vi "Framework Configuration 1.1 Finalize.vi"(8 "error in (no error)":errorcluster, 10 "dsf version (1.1)":T1={"major"=1, "minor"=1, "fix"=0, "build"=""}, 11 "framework configuration 1.1":T2) -> (0 "error out":errorcluster, 2 "final dsf version":T1, 3 "dsf configuration json":string)   [LabVIEW 2017, in "DSF Core.lvlib" / "Configuration Session.lvclass"]
uses:
  Configuration Session.lvclass
  Typedefs/DSF Version Info.ctl
  Framework Configuration 1.1.ctl
  DSF Core.lvlib
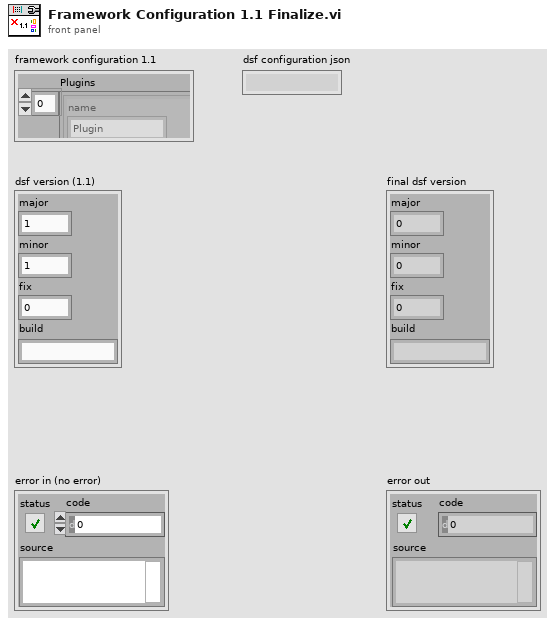
[diagram p1: front panel]
types:
  T1 = typedef "DSF Core.lvlib/DSF Version Info.ctl" = cluster{"major":u32, "minor":u32, "fix":u32, "build":string}
  T2 = typedef "DSF Core.lvlib/Configuration Session.lvclass/Framework Configuration 1.1.ctl" = cluster{"Plugins":cluster{"name":string, "components":string[], "cycle timing":cluster{"priority":u64, "decimation":u64, "offset":u64}, "threads":cluster{"buffer converter settings":cluster{"key":string, "value":string}[], "transceiver settings":cluster{"key":string, "value":string}[], "custom settings":cluster{"key":string, "value":string}[], "processor":i32, "priority offset":i16}[], "Transfer Groups":cluster{"name":string, "direction":enum8{"Tx", "Rx"}, "cycle timing":cluster{"priority":u64, "decimation":u64, "offset":u64}, "thread index":i32, "settings":cluster{"key":string, "value":string}[], "Transfers":cluster{"name":string, "byte order":enum8{"big-endian", "little-endian"}, "settings":cluster{"key":string, "value":string}[], "channels":cluster{"string offset":u64, "string data type":enum8{"Bool", "SGL", "DBL", "I8", "I16", "I32", "I64", "U8", "U16", "U32", "U64"}, "engine data type":enum8{"Bool", "SGL", "DBL", "I8", "I16", "I32", "I64", "U8", "U16", "U32", "U64"}, "name":string, "settings":cluster{"key":string, "value":string}[], "units":string}[]}[], "timeout behavior":enum8{"Increment Late Count", "Throw Error"}}[], "settings":cluster{"key":string, "value":string}[]}[]}
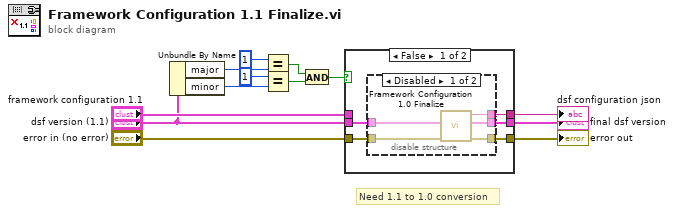
[diagram p0: block diagram]
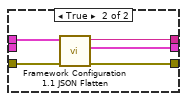
[diagram p3: hidden frame]
diagram:
  # "Need 1.1 to 1.0 conversion"
  n1 = Unbundle By Name("dsf version (1.1)") -> ("major"=w12:u32, "minor"=w13:u32)
  n2 = Equal?(x=u32 1, y=w12) -> (x = y?=w8:bool)
  n3 = Equal?(x=u32 1, y=w13) -> (x = y?=w9:bool)
  n4 = And(x=w8, y=w9) -> (x .and. y?=w7:bool)
  n5 = case shown="False" w7 {
    tunnel: "error in (no error)" -> [w18 w30]
    tunnel: "framework configuration 1.1" -> [_ w29]
    tunnel: [w17 w28] -> w3
    tunnel: "dsf version (1.1)" -> [w14 _]
    tunnel: [w16 w27] -> w4
    tunnel: [w15 w26] -> w1
    frame False {
      n6 = disable-structure shown="Disabled" {
        disable-tunnel: w18 -> [w23 w25]
        disable-tunnel: [w22 w25] -> w17
        disable-tunnel: [w21 _] -> w16
        disable-tunnel: [w20 w24] -> w15
        disable-tunnel: w14 -> [w19 w24]
        frame Disabled {
          n7 = call "Framework Configuration 1.0 Finalize.vi"("error in (no error)"=w23, "dsf version (1.0)"=w19) -> ("error out"=w22:errorcluster, "final dsf version"=w20:T1, "dsf configuration json"=w21:string)  [unwired: 7 in]
        }
        frame Enabled {
        }
      }
    }
    frame True {
      n8 = call "Framework Configuration 1.1 JSON Flatten.vi"("error in (no error)"=w30, "framework configuration 1.1"=w29) -> ("error out"=w28:errorcluster, "dsf version"=w26:T1, "dsf configuration json"=w27:string)  [unwired: 7 in]
    }
  }
  "dsf configuration json" <- w4
  "error out" <- w3
  "final dsf version" <- w1
